vi "Teleop.vi"(10 "Match Info":T1={"Autonomous Elapsed Seconds"=0.0, "TeleOp Elapsed Seconds"=0.0, "Disabled Elapsed Seconds"=0.0, "Visited Autonomous"=FALSE, "Visited TeleOp"=FALSE, "Visited Disabled"=FALSE, "Autonomous Settings"={"Autonomous Style"=enum."Independent", "VI Refnum"=refnum}}, 11 "Call Context":T2) -> ()   [LabVIEW 2015]
doc: "This VI is called for each TeleOp packet received from the DS where the robot is not disabled. It is often used to read from the joysticks and update I/O or to update setpoints for timed control loops. It should complete and return within 20 milliseconds or it may miss DS packets."
uses:
  <vilib>/Rock Robotics/WPI/DriverStation/WPI_DriverStationDerivedRobotMode.ctl
  <vilib>/Rock Robotics/WPI/DriverStation/WPI_DriverStationMatch Info.ctl
  <vilib>/Rock Robotics/WPI/Solenoid/WPI_SolenoidValue.ctl
  <vilib>/Rock Robotics/Network Tables/NT Read Boolean.vi
  <vilib>/Rock Robotics/Network Tables/NT Read Number.vi
  <vilib>/Rock Robotics/WPI/Utilities/WPI_GetSetVariantRefNum.vi
  <vilib>/Rock Robotics/WPI/Solenoid/WPI_SolenoidSetEnum.vi
panel:
  in  "Intake RPM":dbl=1500.0
  in  "error in (no error)":errorcluster
  out "Sample Slider 0":dbl(slide) scale=0.0..5.0
  out "Sample Boolean 1":bool
  out "Sample Boolean 0":bool
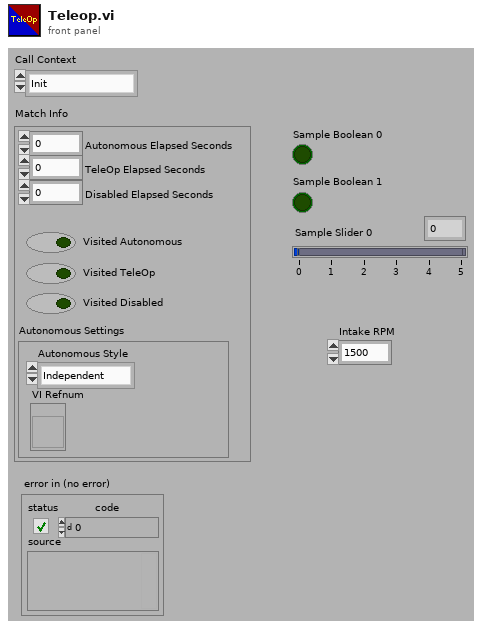
[diagram p1: front panel]
types:
  T1 = typedef "WPI_DriverStationMatch Info.ctl" = cluster{"Autonomous Elapsed Seconds":dbl, "TeleOp Elapsed Seconds":dbl, "Disabled Elapsed Seconds":dbl, "Visited Autonomous":bool, "Visited TeleOp":bool, "Visited Disabled":bool, "Autonomous Settings":cluster{"Autonomous Style":enum16{"Iterative", "Independent"}, "VI Refnum":refnum<vi>}}
  T2 = typedef "WPI_DriverStationDerivedRobotMode.ctl" = enum16{"Init", "Execute", "Stop"}
  T3 = typedef "WPI_SolenoidValue.ctl" = enum16{"Off", "On", "Forward", "Reverse"}
  T4 = typedef "WPI_JoystickDevRef.ctl" = cluster{"Device":T5}
  T5 = typedef "WPI_JoystickDeviceEnum.ctl" = enum16{"USB 0", "USB 1", "USB 2", "USB 3", "USB 4", "USB 5"}
  T6 = cluster{"Axes[0]":dbl, "Axes[1]":dbl, "Axes[2]":dbl, "Axes[3]":dbl, "Axes[4]":dbl, "Axes[5]":dbl, "Axes[6]":dbl, "Axes[7]":dbl, "Axes[8]":dbl}
  T7 = cluster{"Buttons[0]":bool, "Buttons[1]":bool, "Buttons[2]":bool, "Buttons[3]":bool, "Buttons[4]":bool, "Buttons[5]":bool, "Buttons[6]":bool, "Buttons[7]":bool, "Buttons[8]":bool}
  T8 = cluster{"Buttons[0]":bool, "Buttons[1]":bool, "Buttons[2]":bool, "Buttons[3]":bool, "Buttons[4]":bool, "Buttons[5]":bool, "Buttons[6]":bool, "Buttons[7]":bool, "Buttons[8]":bool, "Buttons[9]":bool, "Buttons[10]":bool, "Buttons[11]":bool}
  T9 = cluster{"POVs[0]":i16, "POVs[1]":i16, "POVs[2]":i16, "POVs[3]":i16, "POVs[4]":i16, "POVs[5]":i16, "POVs[6]":i16, "POVs[7]":i16, "POVs[8]":i16}
  T10 = typedef "WPI_SolenoidDevRef.ctl" = cluster{"DevStatus":errorcluster, "Pneumatics Control Module":u8, "Forward Solenoid Channel":T11, "Reverse Solenoid Channel":T11}
  T11 = typedef "WPI_SolenoidChannel.ctl" = enum8{"Solenoid 0", "Solenoid 1", "Solenoid 2", "Solenoid 3", "Solenoid 4", "Solenoid 5", "Solenoid 6", "Solenoid 7", "Invalid"}
  T12 = typedef "WPI_RobotDriveDevRef.ctl" = cluster{"DevStatus":errorcluster, "Motors[]":T13[], "Square Inputs":bool, "Max Output":dbl}
  T13 = typedef "WPI_MotorControlDeviceRef.ctl" = cluster{"DeviceStatus":errorcluster, "Type":T14, "PWM":cluster{"PWM Channel":T15, "DeadBand":T16}, "CAN":cluster{"Device Number":u8, "Control Mode":T17, "Semaphore":T18, "Max Vout":dbl, "TalonSRX Control Mode":T19}, "Invert":bool}
  T14 = typedef "WPI_MotorControlType.ctl" = enum16{"PWM", "CAN", "CANTalonSRX"}
  T15 = typedef "FPGA_DIOPWMChannel.ctl" = enum8{"PWM 0", "PWM 1", "PWM 2", "PWM 3", "PWM 4", "PWM 5", "PWM 6", "PWM 7", "PWM 8", "PWM 9", "PWM MXP 0", "PWM MXP 1", "PWM MXP 2", "PWM MXP 3", "PWM MXP 4", "PWM MXP 5", "PWM MXP 6", "PWM MXP 7", "PWM MXP 8", "PWM MXP 9", "Invalid"}
  T16 = typedef "WPI_PWMDeadband.ctl" = cluster{"Name":string, "maxPositivePwm":i32, "minPositivePwm":i32, "centerPwm":i32, "maxNegativePwm":i32, "minNegativePwm":i32, "angularRange":u16}
  T17 = typedef "WPI_CANJaguar_ControlMode.ctl" = enum8{"Percent VBus", "Current", "Speed", "Position", "Voltage"}
  T18 = typedef "Semaphore RefNum" = refnum<k1>
  T19 = typedef "WPI_CANTalonSRX_APIControlMode.ctl" = enum8{"Percent VBus", "Speed", "Position", "Slave", "Unchanged / Invalid", "Voltage Compensation", "Current", "Motion Profile"}
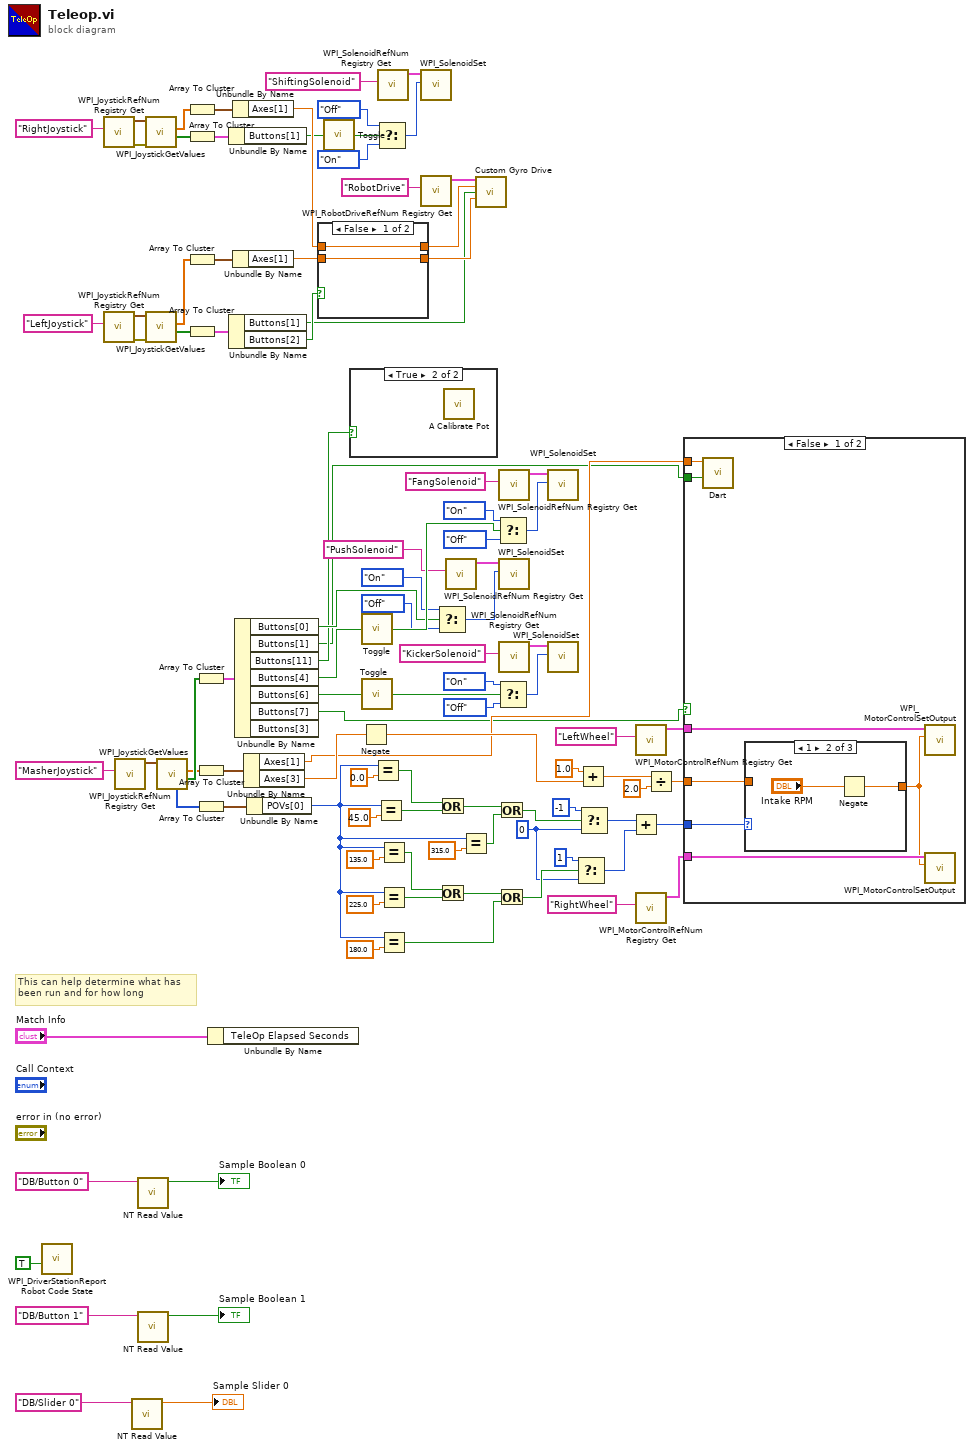
[diagram p0: block diagram]
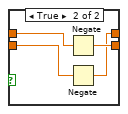
[diagram p2: hidden frame]
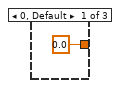
[diagram p4: hidden frame]
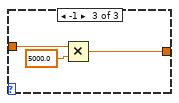
[diagram p5: hidden frame]
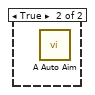
[diagram p6: hidden frame]
diagram:
  w58 = i16 0 ("f")
  # "This can help determine what has\nbeen run and for how long"
  n1 = call <vilib>:"WPI_DriverStationReport Robot Code State.vi"("TeleOp"=TRUE ("Autonomous")) -> ()  [unwired: 10 in, 1 out]
  n2 = call <vilib>:"WPI_JoystickRefNum Registry Get.vi"("refnum name"="RightJoystick") -> ("error out"=w89:errorcluster, "JoystickDevRef"=w88:T4)  [unwired: 9 in]
  n3 = call <vilib>:"WPI_JoystickRefNum Registry Get.vi"("refnum name"="LeftJoystick") -> ("error out"=w82:errorcluster, "JoystickDevRef"=w87:T4)  [unwired: 9 in]
  n4 = call <vilib>:"WPI_JoystickRefNum Registry Get.vi"("refnum name"="MasherJoystick") -> ("JoystickDevRef"=w93:T4)  [unwired: 9 in, 1 out]
  n5 = call-poly <vilib>:"NT Read Value.vi"("Name"="DB/Slider 0" ("refnum name")) -> ("Numeric"=→"Sample Slider 0":dbl)  [unwired: 9 in, 1 out]
  n6 = call-poly <vilib>:"NT Read Value.vi"("Name"="DB/Button 0" ("refnum name")) -> ("Boolean"=→"Sample Boolean 0":bool)  [unwired: 9 in, 1 out]
  n7 = call-poly <vilib>:"NT Read Value.vi"("Name"="DB/Button 1" ("refnum name")) -> ("Boolean"=→"Sample Boolean 1":bool)  [unwired: 9 in, 1 out]
  n8 = call <vilib>:"WPI_JoystickGetValues.vi"("error in (no error)"=w89, "JoystickDevRef"=w88) -> ("Buttons"=w4:bool[], "Axes"=w86:dbl[])  [unwired: 5 in, 3 out]
  n9 = call <vilib>:"WPI_JoystickGetValues.vi"("error in (no error)"=w82, "JoystickDevRef"=w87) -> ("Buttons"=w14:bool[], "Axes"=w85:dbl[])  [unwired: 5 in, 3 out]
  n10 = call <vilib>:"WPI_JoystickGetValues.vi"("JoystickDevRef"=w93) -> ("Buttons"=w92:bool[], "Axes"=w90:dbl[], "POVs"=w57:i16[])  [unwired: 6 in, 2 out]
  n11 = Array To Cluster(array=w86) -> (cluster=w84:T6)
  n12 = Array To Cluster(array=w4) -> (cluster=w3:T7)
  n13 = Array To Cluster(array=w85) -> (cluster=w83:T6)
  n14 = Array To Cluster(array=w14) -> (cluster=w80:T7)
  n15 = Array To Cluster(array=w92) -> (cluster=w81:T8)
  n16 = Array To Cluster(array=w90) -> (cluster=w91:T6)
  n17 = Array To Cluster(array=w57) -> (cluster=w56:T9)
  n18 = Unbundle By Name("Match Info") -> ()  [unwired: 1 out]
  n19 = Unbundle By Name(w3) -> ("Buttons[1]"=w2:bool)
  n20 = Unbundle By Name(w80) -> ("Buttons[1]"=w17:bool, "Buttons[2]"=w20:bool)
  n21 = Unbundle By Name(w84) -> ("Axes[1]"=w79:dbl)
  n22 = Unbundle By Name(w83) -> ("Axes[1]"=w78:dbl)
  n23 = Unbundle By Name(w81) -> ("Buttons[0]"=w31:bool, "Buttons[1]"=w11:bool, "Buttons[11]"=w21:bool, "Buttons[4]"=w48:bool, "Buttons[6]"=w13:bool, "Buttons[7]"=w10:bool)  [unwired: 1 out]
  n24 = Unbundle By Name(w91) -> ("Axes[1]"=w28:dbl, "Axes[3]"=w50:dbl)
  n25 = Unbundle By Name(w56) -> ("POVs[0]"=w55:i16)
  n26 = case shown="False" w20 {
    tunnel: w78 -> [w103 w107]
    tunnel: w79 -> [w104 w108]
    tunnel: [w104 w105] -> w19
    tunnel: [w103 w106] -> w18
    frame False {
    }
    frame True {
      n27 = Negate(x=w108) -> (-x=w106:dbl)
      n28 = Negate(x=w107) -> (-x=w105:dbl)
    }
  }
  n29 = call "Toggle.vi"("Input"=w2) -> ("Output"=w1:bool)
  n30 = case shown="True" w21 {
    frame False {
    }
    frame True {
      n31 = call "A Calibrate Pot.vi"() -> ()  [unwired: 12 in]
    }
  }
  n32 = Negate(x=w50) -> (-x=w51:dbl)
  n33 = call "Toggle.vi"("Input"=w48) -> ("Output"=w47:bool)
  n34 = call "Toggle.vi"("Input"=w13) -> ("Output"=w12:bool)
  n35 = Equal?(x=w55, y=0.0) -> (x = y?=w73:bool)
  n36 = Equal?(x=w55, y=45.0) -> (x = y?=w75:bool)
  n37 = Select(t=WPI_SolenoidValue."Off" ("Value"), s=w1, f=WPI_SolenoidValue."On" ("Value")) -> (s? t:f=w6:T3)
  n38 = call <vilib>:"WPI_SolenoidRefNum Registry Get.vi"("refnum name"="ShiftingSolenoid") -> ("SolenoidDevRef"=w7:T10)  [unwired: 9 in, 1 out]
  n39 = Equal?(x=w55, y=135.0) -> (x = y?=w66:bool)
  n40 = Equal?(x=w55, y=225.0) -> (x = y?=w64:bool)
  n41 = Equal?(x=w55, y=180.0) -> (x = y?=w68:bool)
  n42 = call-poly <vilib>:"WPI_SolenoidSet.vi"("Value"=w6, "SolenoidDevRef"=w7) -> ()  [unwired: 8 in, 2 out]
  n43 = call <vilib>:"WPI_RobotDriveRefNum Registry Get.vi"("refnum name"="RobotDrive") -> ("RobotDriveDevRef"=w27:T12)  [unwired: 9 in, 1 out]
  n44 = Select(t=WPI_SolenoidValue."On" ("Value"), s=w31, f=WPI_SolenoidValue."Off" ("Value")) -> (s? t:f=w39:T3)
  n45 = Or(x=w73, y=w75) -> (x .or. y?=w77:bool)
  n46 = Or(x=w66, y=w64) -> (x .or. y?=w62:bool)
  n47 = call <vilib>:"WPI_SolenoidRefNum Registry Get.vi"("refnum name"="PushSolenoid") -> ("SolenoidDevRef"=w38:T10)  [unwired: 9 in, 1 out]
  n48 = Equal?(x=w55, y=315.0) -> (x = y?=w71:bool)
  n49 = call "Custom Gyro Drive.vi"("RobotDriveDevRef"=w27, "Left Joystick"=w19, "Gyro Correction"=w17, "Right Joystick"=w18) -> ()  [unwired: 7 in, 5 out]
  n50 = Or(x=w77, y=w71) -> (x .or. y?=w49:bool)
  n51 = Or(x=w62, y=w68) -> (x .or. y?=w59:bool)
  n52 = Select(t=WPI_SolenoidValue."On" ("Value"), s=w47, f=WPI_SolenoidValue."Off" ("Value")) -> (s? t:f=w44:T3)
  n53 = Select(t=WPI_SolenoidValue."On" ("Value"), s=w12, f=WPI_SolenoidValue."Off" ("Value")) -> (s? t:f=w34:T3)
  n54 = call <vilib>:"WPI_SolenoidRefNum Registry Get.vi"("refnum name"="FangSolenoid") -> ("SolenoidDevRef"=w45:T10)  [unwired: 9 in, 1 out]
  n55 = call-poly <vilib>:"WPI_SolenoidSet.vi"("Value"=w39, "SolenoidDevRef"=w38) -> ()  [unwired: 8 in, 2 out]
  n56 = call <vilib>:"WPI_SolenoidRefNum Registry Get.vi"("refnum name"="KickerSolenoid") -> ("SolenoidDevRef"=w35:T10)  [unwired: 9 in, 1 out]
  n57 = call-poly <vilib>:"WPI_SolenoidSet.vi"("Value"=w44, "SolenoidDevRef"=w45) -> ()  [unwired: 8 in, 2 out]
  n58 = call-poly <vilib>:"WPI_SolenoidSet.vi"("Value"=w34, "SolenoidDevRef"=w35) -> ()  [unwired: 8 in, 2 out]
  n59 = Select(t=i16 1, s=w59, f=w58) -> (s? t:f=w60:i16)
  n60 = Add(x=1.0, y=w51) -> (x+y=w53:dbl)
  n61 = Select(t=i16 -1, s=w49, f=w58) -> (s? t:f=w69:i16)
  n62 = Add(x=w69, y=w60) -> (x+y=w30:i16)
  n63 = call <vilib>:"WPI_MotorControlRefNum Registry Get.vi"("refnum name"="LeftWheel") -> ("MotorControlDevRef"=w23:T13)  [unwired: 9 in, 1 out]
  n64 = call <vilib>:"WPI_MotorControlRefNum Registry Get.vi"("refnum name"="RightWheel") -> ("MotorControlDevRef"=w22:T13)  [unwired: 9 in, 1 out]
  n65 = Divide(x=w53, y=2.0) -> (x/y=w29:dbl)
  n66 = case shown="False" w10 {
    tunnel: w30 -> [w115 _]
    tunnel: w29 -> [w114 _]
    tunnel: w28 -> [w113 _]
    tunnel: w11 -> [w112 _]
    tunnel: w23 -> [w111 _]
    tunnel: w22 -> [w110 _]
    frame False {
      n67 = call "Dart.vi"("Enable Drive"=w112, "Power Input"=w113) -> ()  [unwired: 10 in]
      n68 = case shown="1" w115 {
        tunnel: [0.0 w117 w119] -> w109
        tunnel: w114 -> [_ _ w120]
        frame 0, Default {
        }
        frame 1 {
          n69 = Negate(x="Intake RPM") -> (-x=w117:dbl)
        }
        frame -1 {
          n70 = Multiply(x=w120, y=5000.0) -> (x*y=w119:dbl)
        }
      }
      n71 = call <vilib>:"WPI_MotorControlSetOutput.vi"("Output"=w109, "MotorControlDevRef"=w111) -> ()  [unwired: 7 in, 3 out]
      n72 = call <vilib>:"WPI_MotorControlSetOutput.vi"("Output"=w109, "MotorControlDevRef"=w110) -> ()  [unwired: 7 in, 3 out]
    }
    frame True {
      n73 = call "A Auto Aim.vi"() -> ()  [unwired: 12 in]
    }
  }
